vi "Begin.vi"(8 "error in":errorcluster) -> (0 "error out":errorcluster)   [LabVIEW 2019]
doc: "Called before other user functions, this VI is expected to open initial I/O refnums, load in file data, and do all program initialization. Notice that the <B>error out</B> terminal is simply used for data flow. Wiring it to other structures or subVIs ensures that this VI runs first."
uses:
  <vilib>/Rock Robotics/WPI/SafetyOutput/WPI_SafetyOutputConfigMenu.ctl
  <vilib>/Rock Robotics/WPI/DriverStation/WPI_DriverStationRobotMode2.ctl
  <vilib>/Rock Robotics/SystemInterfaces/DIO/FPGA_DIOChannel.ctl
  <vilib>/Rock Robotics/WPI/Encoder/WPI_EncoderType.ctl
  <vilib>/Rock Robotics/WPI/Joystick/WPI_JoystickDeviceEnum.ctl
  <vilib>/Rock Robotics/Network Tables/NT Write Boolean.vi
  <vilib>/Rock Robotics/Network Tables/NT Write Number.vi
  <vilib>/Rock Robotics/WPI/Switch/WPI_SwitchOpenLimit.vi
  <vilib>/Rock Robotics/WPI/Counter/WPI_CounterDigitalInputToDigitalSource.vi
  Robot Global Data.vi
  <vilib>/Rock Robotics/WPI/RobotDrive/WPI_RobotDriveOpen2MotorWithExistingMotors.vi
  <vilib>/Rock Robotics/Network Tables/NT Write String Array.vi
  <vilib>/Rock Robotics/SystemInterfaces/i2clib/i2c_bus.ctl
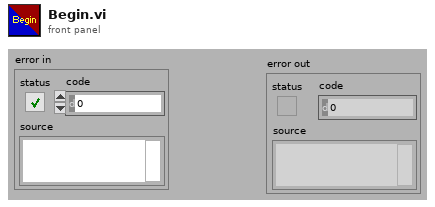
[diagram p1: front panel]
types:
  T1 = typedef "WPI_JoystickDeviceEnum.ctl" = enum16{"USB 0", "USB 1", "USB 2", "USB 3", "USB 4", "USB 5"}
  T2 = typedef "WPI_JoystickDevRef.ctl" = cluster{"Device":T1}
  T3 = typedef "WPI_DriverStationRobotMode2.ctl" = enum16{"Autonomous Disabled", "Autonomous Enabled", "Teleop Disabled", "Teleop Enabled", "Disconnected", "Finish", "Test Disabled", "Test Enabled", "Emergency Stopped"}
  T4 = typedef "WPI_SafetyOutputConfigMenu.ctl" = enum16{"Enable", "Disable"}
  T5 = typedef "WPI_MotorControlDeviceRef.ctl" = cluster{"DeviceStatus":errorcluster, "Type":T6, "PWM":cluster{"PWM Channel":T7, "DeadBand":T8}, "CAN":cluster{"Device Number":u8, "SetOutput VI Ref":variant, "GetOutput VI Ref":variant, "Enable VI Ref":variant, "Disable VI Ref":variant, "Data":variant}, "Invert":bool, "DIO PWM":cluster{"PWM \"Enable\" Channel":T7, "DIOChannel":T9, "PWM Rate":dbl}}
  T6 = typedef "WPI_MotorControlType.ctl" = enum16{"PWM", "CAN", "DIO PWM"}
  T7 = typedef "FPGA_DIOPWMChannel.ctl" = enum8{"PWM 0", "PWM 1", "PWM 2", "PWM 3", "PWM 4", "PWM 5", "PWM 6", "PWM 7", "PWM 8", "PWM 9", "PWM MXP 0", "PWM MXP 1", "PWM MXP 2", "PWM MXP 3", "PWM MXP 4", "PWM MXP 5", "PWM MXP 6", "PWM MXP 7", "PWM MXP 8", "PWM MXP 9", "Invalid"}
  T8 = typedef "WPI_PWMDeadband.ctl" = cluster{"Name":string, "maxPositivePwm":i32, "minPositivePwm":i32, "centerPwm":i32, "maxNegativePwm":i32, "minNegativePwm":i32, "angularRange":u16}
  T9 = typedef "FPGA_DIOChannel.ctl" = enum8{"DIO 0", "DIO 1", "DIO 2", "DIO 3", "DIO 4", "DIO 5", "DIO 6", "DIO 7", "DIO 8", "DIO 9", "DIO MXP 0", "DIO MXP 1", "DIO MXP 2", "DIO MXP 3", "DIO MXP 4", "DIO MXP 5", "DIO MXP 6", "DIO MXP 7", "DIO MXP 8", "DIO MXP 9", "DIO MXP 10", "DIO MXP 11", "DIO MXP 12", "DIO MXP 13", "DIO MXP 14", "DIO MXP 15", "SPI Port CS1", "SPI Port CS2", "SPI Port CS3", "SPI Port MISO", "SPI Port MOSI", "Invalid"}
  T10 = typedef "WPI_RobotDriveDevRef.ctl" = cluster{"DevStatus":errorcluster, "Motors[]":T5[], "Square Inputs":bool, "Max Output":dbl}
  T11 = typedef "i2c_bus.ctl" = enum16{"I2C On-Board", "I2C MXP", "Invalid"}
  T12 = typedef "WPI_SwitchDevRef.ctl" = cluster{"DevStatus":errorcluster, "DIO Channel":T9, "CntIndex":T13, "Normally Closed":bool}
  T13 = typedef "FPGA_CounterCtrSystemIndex.ctl" = enum8{"Ctr 0", "Ctr 1", "Ctr 2", "Ctr 3", "Ctr 4", "Ctr 5", "Ctr 6", "Ctr 7", "Invalid"}
  T14 = typedef "WPI_EncoderType.ctl" = enum16{"1x", "2x", "4x"}
  T15 = typedef "WPI_DigitalInputDevRef.ctl" = cluster{"DevStatus":errorcluster, "DIO Channel":T9}
  T16 = typedef "FPGA_CounterEncoderSourceConvertionLVSourceType.ctl" = cluster{"DevStatus":errorcluster, "AnalogTriggerMode?":bool, "DigitalMode":cluster{"DIO Channel":T17}, "AnalogTriggerMode":cluster{"AnalogTriggerIndex":T18, "OutputType":T19}}
  T17 = typedef "FPGA_DIODigitalSourceChannel.ctl" = enum8{"DIO 0", "DIO 1", "DIO 2", "DIO 3", "DIO 4", "DIO 5", "DIO 6", "DIO 7", "DIO 8", "DIO 9", "DIO MXP 0", "DIO MXP 1", "DIO MXP 2", "DIO MXP 3", "DIO MXP 4", "DIO MXP 5", "DIO MXP 6", "DIO MXP 7", "DIO MXP 8", "DIO MXP 9", "DIO MXP 10", "DIO MXP 11", "DIO MXP 12", "DIO MXP 13", "DIO MXP 14", "DIO MXP 15", "SPI Port CS1", "SPI Port CS2", "SPI Port CS3", "SPI Port MISO", "SPI Port MOSI", "Disabled"}
  T18 = typedef "FPGA_AnalogTriggerIndex.ctl" = enum8{"Trig 0", "Trig 1", "Trig 2", "Trig 3", "Trig 4", "Trig 5", "Trig 6", "Trig 7", "Invalid"}
  T19 = typedef "FPGA_AnalogTriggerOutType.ctl" = enum16{"InWindow", "TriggerState", "Rising", "Falling"}
  T20 = typedef "WPI_EncoderDevRef.ctl" = cluster{"DevStatus":errorcluster, "EncoderIndex":T21, "CounterIndex":T13, "DistancePerCount":dbl, "Decoding Type":T14}
  T21 = typedef "FPGA_EncoderIdx.ctl" = enum8{"Enc 0", "Enc 1", "Enc 2", "Enc 3", "Enc 4", "Enc 5", "Enc 6", "Enc 7", "Invalid"}
  T22 = typedef "WPI_ServoDeviceRef.ctl" = cluster{"DeviceStatus":errorcluster, "PWM Channel":T7, "DeadBand":T8}
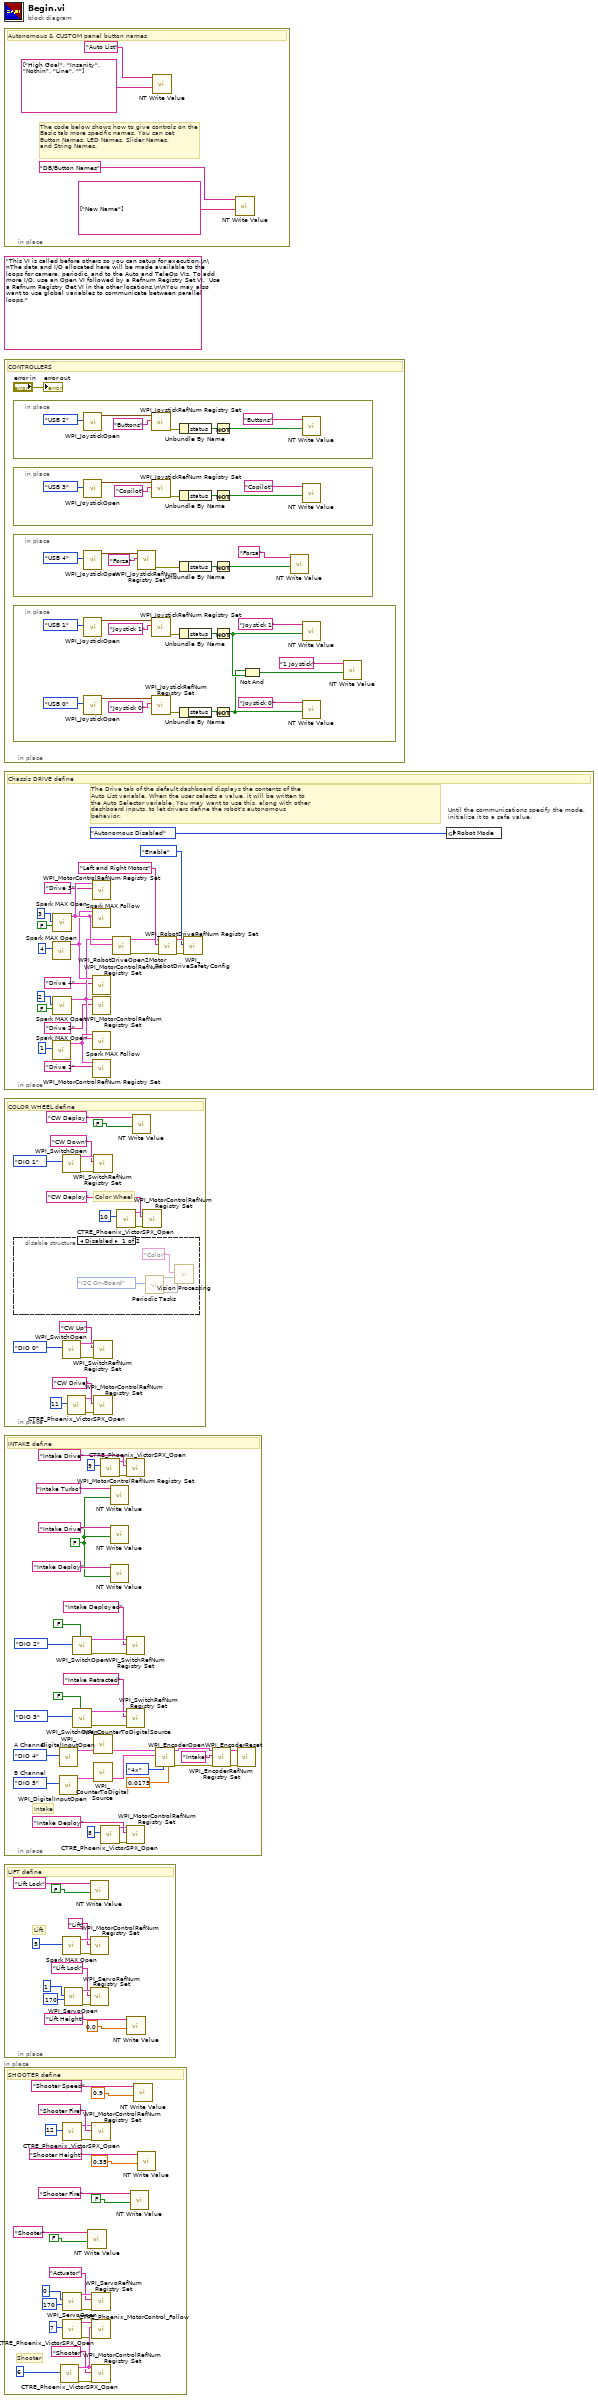
[diagram p0: block diagram]
diagram:
  (unwired) "This VI is called before others so you can setup for execution.\n\nThe data and I/O allocated here will be made available to the loops for camera, periodic, and to the Auto and TeleOp VIs. To add more I/O, use an Open VI followed by a Refnum Registry Set VI.  Use a Refnum Registry Get VI in the other locations.\n\nYou may also want to use global variables to communicate between parallel loops."
  n1 = in-place {
    # "The code below shows how to give controls on the\nBasic tab more specific names. You can set\nButton Names, LED Names, Slider Names,\nand String Names."
    # "Autonomous & CUSTOM panel button names"
    n2 = call-poly <vilib>:"NT Write Value.vi"("String Array"=string[] ["High Goal", "Insanity", "Nothin", "Line", ""], "Name"="Auto List") -> ()  [unwired: 9 in, 1 out]
    n3 = call-poly <vilib>:"NT Write Value.vi"("String Array"=string[] ["New Name"], "Name"="DB/Button Names") -> ()  [unwired: 9 in, 1 out]
  }
  n4 = in-place {
    # "CONTROLLERS"
    n5 = in-place {
      n6 = call <vilib>:"WPI_JoystickOpen.vi"("JoystickDevice"=WPI_JoystickDeviceEnum."USB 2") -> ("JoystickDevRef"=w11:T2)  [unwired: 10 in]
      n7 = call <vilib>:"WPI_JoystickRefNum Registry Set.vi"("refnum name"="Buttons", "JoystickDevRef"=w11) -> ("error out"=w7:errorcluster)  [unwired: 8 in, 1 out]
      n8 = Unbundle By Name(w7) -> ("status"=w6:bool)
      n9 = Not(x=w6) -> (.not. x?=w8:bool)
      n10 = call-poly <vilib>:"NT Write Value.vi"("Boolean"=w8, "Name"="Buttons") -> ()  [unwired: 9 in, 1 out]
    }
    n11 = in-place {
      n12 = call <vilib>:"WPI_JoystickOpen.vi"("JoystickDevice"=WPI_JoystickDeviceEnum."USB 3") -> ("JoystickDevRef"=w18:T2)  [unwired: 10 in]
      n13 = call <vilib>:"WPI_JoystickRefNum Registry Set.vi"("refnum name"="Copilot", "JoystickDevRef"=w18) -> ("error out"=w14:errorcluster)  [unwired: 8 in, 1 out]
      n14 = Unbundle By Name(w14) -> ("status"=w13:bool)
      n15 = Not(x=w13) -> (.not. x?=w15:bool)
      n16 = call-poly <vilib>:"NT Write Value.vi"("Boolean"=w15, "Name"="Copilot") -> ()  [unwired: 9 in, 1 out]
    }
    n17 = in-place {
      n18 = call <vilib>:"WPI_JoystickOpen.vi"("JoystickDevice"=WPI_JoystickDeviceEnum."USB 4") -> ("JoystickDevRef"=w24:T2)  [unwired: 10 in]
      n19 = call <vilib>:"WPI_JoystickRefNum Registry Set.vi"("refnum name"="Forza", "JoystickDevRef"=w24) -> ("error out"=w22:errorcluster)  [unwired: 8 in, 1 out]
      n20 = Unbundle By Name(w22) -> ("status"=w21:bool)
      n21 = Not(x=w21) -> (.not. x?=w20:bool)
      n22 = call-poly <vilib>:"NT Write Value.vi"("Boolean"=w20, "Name"="Forza") -> ()  [unwired: 9 in, 1 out]
    }
    n23 = in-place {
      n24 = call <vilib>:"WPI_JoystickOpen.vi"("JoystickDevice"=WPI_JoystickDeviceEnum."USB 1") -> ("JoystickDevRef"=w36:T2)  [unwired: 10 in]
      n25 = call <vilib>:"WPI_JoystickOpen.vi"("JoystickDevice"=WPI_JoystickDeviceEnum."USB 0") -> ("JoystickDevRef"=w39:T2)  [unwired: 10 in]
      n26 = call <vilib>:"WPI_JoystickRefNum Registry Set.vi"("refnum name"="Joystick 1", "JoystickDevRef"=w36) -> ("error out"=w42:errorcluster)  [unwired: 8 in, 1 out]
      n27 = call <vilib>:"WPI_JoystickRefNum Registry Set.vi"("refnum name"="Joystick 0", "JoystickDevRef"=w39) -> ("error out"=w41:errorcluster)  [unwired: 8 in, 1 out]
      n28 = Unbundle By Name(w42) -> ("status"=w32:bool)
      n29 = Unbundle By Name(w41) -> ("status"=w33:bool)
      n30 = Not(x=w32) -> (.not. x?=w29:bool)
      n31 = Not(x=w33) -> (.not. x?=w27:bool)
      n32 = Not And(1:w29, 2:w27) -> (0:w31:bool)
      n33 = call-poly <vilib>:"NT Write Value.vi"("Boolean"=w29, "Name"="Joystick 1") -> ()  [unwired: 9 in, 1 out]
      n34 = call-poly <vilib>:"NT Write Value.vi"("Boolean"=w27, "Name"="Joystick 0") -> ()  [unwired: 9 in, 1 out]
      n35 = call-poly <vilib>:"NT Write Value.vi"("Boolean"=w31, "Name"="1 Joystick") -> ()  [unwired: 9 in, 1 out]
    }
    "error out" <- "error in"
  }
  n36 = in-place {
    # "The Drive tab of the default dashboard displays the contents of the\nAuto List variable. When the user selects a value, it will be written to\nthe Auto Selector variable. You may want to use this, along with other\ndashboard inputs, to let drivers define the robot's autonomous\nbehavior."
    # "Until the communications specify the mode,\ninitialize it to a safe value."
    # "Chassis DRIVE define"
    n37 = call <vilib>:"Spark MAX Open.vi"("Device Number"=4) -> ("MotorControlDeviceRef"=w51:T5)  [unwired: 9 in, 1 out]
    n38 = call <vilib>:"Spark MAX Open.vi"("Device Number"=1) -> ("MotorControlDeviceRef"=w50:T5)  [unwired: 9 in, 1 out]
    n39 = call <vilib>:"Spark MAX Open.vi"("Invert"=FALSE ("RightMotorInverted"), "Device Number"=3) -> ("MotorControlDeviceRef"=w52:T5)  [unwired: 8 in, 1 out]
    n40 = call <vilib>:"Spark MAX Open.vi"("Invert"=FALSE ("LeftMotorInverted"), "Device Number"=2) -> ("MotorControlDeviceRef"=w49:T5)  [unwired: 8 in, 1 out]
    n41 = call <vilib>:"WPI_MotorControlRefNum Registry Set.vi"("refnum name"="Drive 3", "MotorControlDevRef"=w52) -> ()  [unwired: 8 in, 2 out]
    n42 = call <vilib>:"Spark MAX Follow.vi"("Master Controller"=w52, "MotorControlDeviceRef"=w51) -> ()  [unwired: 8 in, 2 out]
    n43 = call <vilib>:"WPI_MotorControlRefNum Registry Set.vi"("refnum name"="Drive 4", "MotorControlDevRef"=w51) -> ()  [unwired: 8 in, 2 out]
    n44 = call <vilib>:"WPI_MotorControlRefNum Registry Set.vi"("refnum name"="Drive 2", "MotorControlDevRef"=w49) -> ()  [unwired: 8 in, 2 out]
    n45 = call <vilib>:"Spark MAX Follow.vi"("Master Controller"=w49, "MotorControlDeviceRef"=w50) -> ()  [unwired: 8 in, 2 out]
    n46 = call <vilib>:"WPI_MotorControlRefNum Registry Set.vi"("refnum name"="Drive 1", "MotorControlDevRef"=w50) -> ()  [unwired: 8 in, 2 out]
    n47 = call-poly <vilib>:"WPI_RobotDriveOpen2Motor.vi"("Right Motor Dev Ref"=w52, "Left Motor Dev Ref"=w49) -> ("error out"=w43:errorcluster, "RobotDriveDevRef"=w55:T10)  [unwired: 8 in]
    n48 = call <vilib>:"WPI_RobotDriveRefNum Registry Set.vi"("error in (no error)"=w43, "refnum name"="Left and Right Motors", "RobotDriveDevRef"=w55) -> ("error out"=w44:errorcluster, "RobotDriveDevRef"=w62:T10)  [unwired: 1 in, 6 out]
    n49 = call <vilib>:"WPI_RobotDriveSafetyConfig.vi"("error in (no error)"=w44, "mode"=WPI_SafetyOutputConfigMenu."Enable", "RobotDriveDevRef"=w62) -> ()  [unwired: 7 in, 2 out]
    n50 = global write "Robot Global Data.vi" "Robot Mode"(WPI_DriverStationRobotMode2."Autonomous Disabled" ("Robot Mode")) -> ()
  }
  n51 = in-place {
    # "Color Wheel"
    # "COLOR WHEEL define"
    n52 = disable-structure shown="Disabled" {
      frame Disabled {
        n53 = call "Periodic Tasks.vi"(10:i2c_bus."I2C On-Board" ("I2C Bus")) -> (0:w85, 3:w84)  [unwired: 9 in]
        n54 = call "Vision Processing.vi"("error in (no error)"=w85, "refnum name"="Color", "ColorSensorDevRef"=w84) -> ()  [unwired: 7 in, 2 out]
      }
      frame Enabled {
      }
    }
    n55 = call-poly <vilib>:"WPI_SwitchOpen.vi"("DIO Channel"=FPGA_DIOChannel."DIO 1") -> ("error out"=w69:errorcluster, "SwitchDevRef"=w68:T12)  [unwired: 9 in]
    n56 = call-poly <vilib>:"WPI_SwitchOpen.vi"("DIO Channel"=FPGA_DIOChannel."DIO 0") -> ("error out"=w72:errorcluster, "SwitchDevRef"=w71:T12)  [unwired: 9 in]
    n57 = call <vilib>:"CTRE_Phoenix_VictorSPX_Open.vi"("Device Number"=11) -> ("error out"=w74:errorcluster, "CAN Talon SRX Ref"=w75:T5)  [unwired: 9 in]
    n58 = call <vilib>:"WPI_SwitchRefNum Registry Set.vi"("error in (no error)"=w69, "refnum name"="CW Down", "SwitchDevRef"=w68) -> ()  [unwired: 7 in, 2 out]
    n59 = call <vilib>:"WPI_SwitchRefNum Registry Set.vi"("error in (no error)"=w72, "refnum name"="CW Up", "SwitchDevRef"=w71) -> ()  [unwired: 7 in, 2 out]
    n60 = call <vilib>:"WPI_MotorControlRefNum Registry Set.vi"("error in (no error)"=w74, "refnum name"="CW Drive", "MotorControlDevRef"=w75) -> ()  [unwired: 7 in, 2 out]
    n61 = call <vilib>:"CTRE_Phoenix_VictorSPX_Open.vi"("Device Number"=10) -> ("error out"=w78:errorcluster, "CAN Talon SRX Ref"=w79:T5)  [unwired: 9 in]
    n62 = call-poly <vilib>:"NT Write Value.vi"("Boolean"=FALSE, "Name"="CW Deploy") -> ()  [unwired: 9 in, 1 out]
    n63 = call <vilib>:"WPI_MotorControlRefNum Registry Set.vi"("error in (no error)"=w78, "refnum name"="CW Deploy", "MotorControlDevRef"=w79) -> ()  [unwired: 7 in, 2 out]
  }
  n64 = in-place {
    w90 = FPGA_DIOChannel."DIO 5"  # B Channel
    w89 = FPGA_DIOChannel."DIO 4"  # A Channel
    w86 = FALSE ("Boolean")
    # "Intake"
    # "INTAKE define"
    n65 = call <vilib>:"WPI_DigitalInputOpen.vi"("DIO Channel"=w89) -> ("DigitalInputDevRef"=w87:T15)  [unwired: 1 in, 9 out]
    n66 = call <vilib>:"WPI_DigitalInputOpen.vi"("DIO Channel"=w90) -> ("DigitalInputDevRef"=w88:T15)  [unwired: 1 in, 9 out]
    n67 = call-poly <vilib>:"WPI_SwitchOpen.vi"("Normally Closed"=FALSE, "DIO Channel"=FPGA_DIOChannel."DIO 2") -> ("error out"=w99:errorcluster, "SwitchDevRef"=w98:T12)  [unwired: 8 in]
    n68 = call-poly <vilib>:"WPI_SwitchOpen.vi"("Normally Closed"=FALSE, "DIO Channel"=FPGA_DIOChannel."DIO 3") -> ("error out"=w95:errorcluster, "SwitchDevRef"=w94:T12)  [unwired: 8 in]
    n69 = call-poly <vilib>:"WPI_CounterToDigitalSource.vi"("DigitalInputDevRef"=w87) -> ("Digital Source"=w119:T16)  [unwired: 6 out]
    n70 = call-poly <vilib>:"WPI_CounterToDigitalSource.vi"("DigitalInputDevRef"=w88) -> ("Digital Source"=w120:T16)  [unwired: 6 out]
    n71 = call <vilib>:"CTRE_Phoenix_VictorSPX_Open.vi"("Device Number"=9) -> ("error out"=w103:errorcluster, "CAN Talon SRX Ref"=w104:T5)  [unwired: 9 in]
    n72 = call <vilib>:"CTRE_Phoenix_VictorSPX_Open.vi"("Device Number"=8) -> ("error out"=w108:errorcluster, "CAN Talon SRX Ref"=w109:T5)  [unwired: 9 in]
    n73 = call-poly <vilib>:"NT Write Value.vi"("Boolean"=w86, "Name"="Intake Turbo") -> ()  [unwired: 9 in, 1 out]
    n74 = call-poly <vilib>:"NT Write Value.vi"("Boolean"=w86, "Name"="Intake Drive") -> ()  [unwired: 9 in, 1 out]
    n75 = call-poly <vilib>:"NT Write Value.vi"("Boolean"=w86, "Name"="Intake Deploy") -> ()  [unwired: 9 in, 1 out]
    n76 = call <vilib>:"WPI_MotorControlRefNum Registry Set.vi"("error in (no error)"=w103, "refnum name"="Intake Drive", "MotorControlDevRef"=w104) -> ()  [unwired: 7 in, 2 out]
    n77 = call <vilib>:"WPI_SwitchRefNum Registry Set.vi"("error in (no error)"=w99, "refnum name"="Intake Deployed", "SwitchDevRef"=w98) -> ()  [unwired: 7 in, 2 out]
    n78 = call <vilib>:"WPI_SwitchRefNum Registry Set.vi"("error in (no error)"=w95, "refnum name"="Intake Retracted", "SwitchDevRef"=w94) -> ()  [unwired: 7 in, 2 out]
    n79 = call <vilib>:"WPI_MotorControlRefNum Registry Set.vi"("error in (no error)"=w108, "refnum name"="Intake Deploy", "MotorControlDevRef"=w109) -> ()  [unwired: 7 in, 2 out]
    n80 = call <vilib>:"WPI_EncoderOpen.vi"("DistancePerCount"=0.0175, "Decoding Type"=WPI_EncoderType."4x", "BSource"=w120, "ASource"=w119) -> ("error out"=w118:errorcluster, "EncoderDevRef"=w117:T20)  [unwired: 4 in, 2 out]
    n81 = call <vilib>:"WPI_EncoderRefNum Registry Set.vi"("error in (no error)"=w118, "refnum name"="Intake", "EncoderDevRef"=w117) -> ("error out"=w115:errorcluster, "EncoderDevRef"=w114:T20)  [unwired: 7 in]
    n82 = call <vilib>:"WPI_EncoderReset.vi"("error in (no error)"=w115, "EncoderDevRef"=w114) -> ()  [unwired: 8 in, 2 out]
  }
  n83 = in-place {
    # "Lift"
    # "LIFT define"
    n84 = call <vilib>:"Spark MAX Open.vi"("Device Number"=u8 5) -> ("error out"=w133:errorcluster, "MotorControlDeviceRef"=w132:T5)  [unwired: 9 in]
    n85 = call <vilib>:"WPI_ServoOpen.vi"("Angular Range"=u16 170, "PWM Channel"=1) -> ("error out"=w127:errorcluster, "ServoDeviceRef"=w129:T22)  [unwired: 8 in]
    n86 = call-poly <vilib>:"NT Write Value.vi"("Boolean"=FALSE, "Name"="Lift Lock") -> ()  [unwired: 9 in, 1 out]
    n87 = call <vilib>:"WPI_MotorControlRefNum Registry Set.vi"("error in (no error)"=w133, "refnum name"="Lift", "MotorControlDevRef"=w132) -> ()  [unwired: 7 in, 2 out]
    n88 = call <vilib>:"WPI_ServoRefNum Registry Set.vi"("error in (no error)"=w127, "refnum name"="Lift Lock", "ServoDeviceRef"=w129) -> ()  [unwired: 7 in, 2 out]
    n89 = call-poly <vilib>:"NT Write Value.vi"("Numeric"=0.0, "Name"="Lift Height") -> ()  [unwired: 9 in, 1 out]
  }
  n90 = in-place {
    # "Shooter"
    # "SHOOTER define"
    n91 = call <vilib>:"CTRE_Phoenix_VictorSPX_Open.vi"("Device Number"=6) -> ("error out"=w148:errorcluster, "CAN Talon SRX Ref"=w151:T5)  [unwired: 9 in]
    n92 = call <vilib>:"CTRE_Phoenix_VictorSPX_Open.vi"("Device Number"=12) -> ("error out"=w143:errorcluster, "CAN Talon SRX Ref"=w144:T5)  [unwired: 9 in]
    n93 = call <vilib>:"WPI_ServoOpen.vi"("Angular Range"=u16 170, "PWM Channel"=0) -> ("error out"=w147:errorcluster, "ServoDeviceRef"=w154:T22)  [unwired: 8 in]
    n94 = call <vilib>:"CTRE_Phoenix_VictorSPX_Open.vi"("Device Number"=7) -> ("error out"=w149:errorcluster, "CAN Talon SRX Ref"=w157:T5)  [unwired: 9 in]
    n95 = call-poly <vilib>:"NT Write Value.vi"("Boolean"=FALSE, "Name"="Shooter") -> ()  [unwired: 9 in, 1 out]
    n96 = call <vilib>:"WPI_MotorControlRefNum Registry Set.vi"("error in (no error)"=w143, "refnum name"="Shooter Fire", "MotorControlDevRef"=w144) -> ()  [unwired: 7 in, 2 out]
    n97 = call <vilib>:"WPI_ServoRefNum Registry Set.vi"("error in (no error)"=w147, "refnum name"="Actuator", "ServoDeviceRef"=w154) -> ()  [unwired: 7 in, 2 out]
    n98 = call <vilib>:"CTRE_Phoenix_MotorControl_Follow.vi"("error in (no error)"=w149, "Master Controller to Follow"=w151, "PhoenixMotorControlDevRef"=w157) -> ()  [unwired: 7 in, 2 out]
    n99 = call <vilib>:"WPI_MotorControlRefNum Registry Set.vi"("error in (no error)"=w148, "refnum name"="Shooter", "MotorControlDevRef"=w151) -> ()  [unwired: 7 in, 2 out]
    n100 = call-poly <vilib>:"NT Write Value.vi"("Boolean"=FALSE, "Name"="Shooter Fire") -> ()  [unwired: 9 in, 1 out]
    n101 = call-poly <vilib>:"NT Write Value.vi"("Numeric"=0.9, "Name"="Shooter Speed") -> ()  [unwired: 9 in, 1 out]
    n102 = call-poly <vilib>:"NT Write Value.vi"("Numeric"=0.35, "Name"="Shooter Height") -> ()  [unwired: 9 in, 1 out]
  }
